vi "ReadSummaryResults.vi"(8 "error in (no error)":errorcluster, 11 "Path":path) -> (0 "error out":errorcluster, 3 "Results":dbl[][](array[numeric]))   [LabVIEW 2014]
uses:
  Excel(ActiveX)/enumOpenOrCreate.ctl
  Excel(ActiveX)/Excel(ActiveX).lvlib
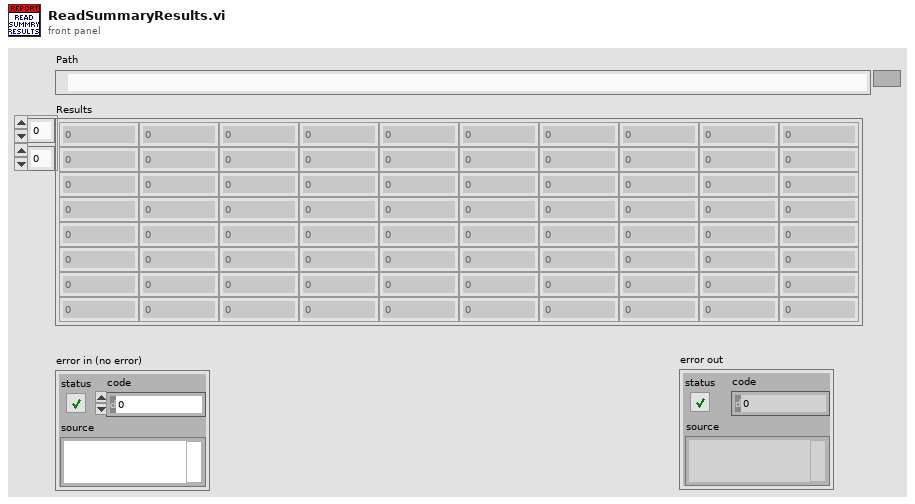
[diagram p1: front panel]
types:
  T1 = typedef "Excel(ActiveX).lvlib/enumOpenOrCreate.ctl" = enum16{"open", "open or create", "create from template"}
  T2 = typedef "Excel(ActiveX).lvlib/ExcelActiveX.ctl" = cluster{"Excel._Application":refnum<k7>, "Application open at start":bool, "Excel._Worksheet":refnum<k7>, "Workbook open at start":bool, "Excel._Workbook":refnum<k7>, "Workbook Path":path, "Worksheet Name":string, "Row":u32, "Col":u32, "Cell":string, "Workbook Name":string}
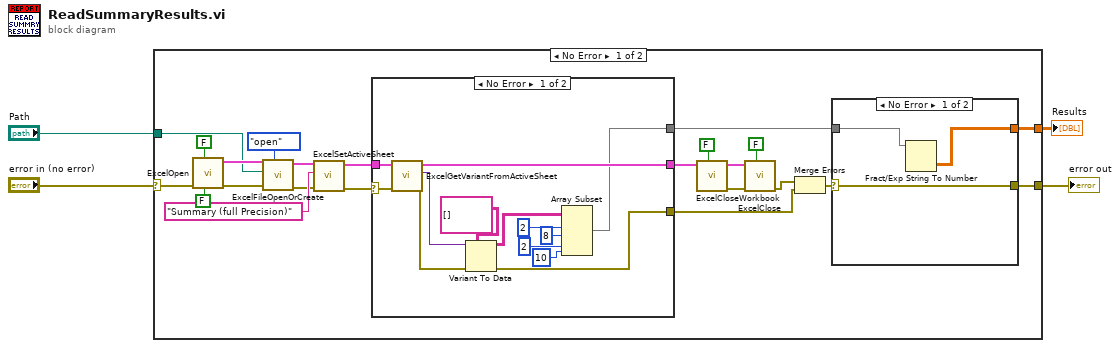
[diagram p0: block diagram]
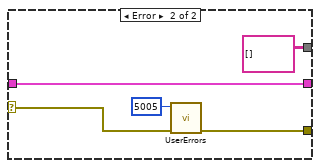
[diagram p2: hidden frame]
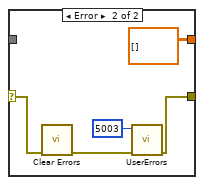
[diagram p3: hidden frame]
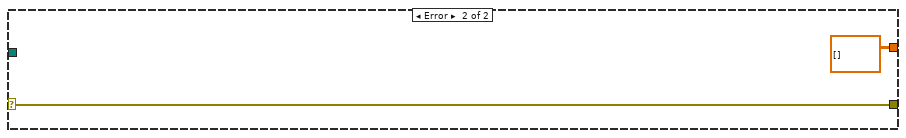
[diagram p4: hidden frame]
diagram:
  n1 = case shown="No Error" "error in (no error)" {
    selector: "error in (no error)" -> [w25 w55]
    tunnel: [w14 w55] -> w3
    tunnel: "Path" -> [w21 _]
    tunnel: [w9 dbl[][] []] -> w1
    frame No Error {
      n2 = call "ExcelOpen.vi"("Run Minimized (f)"=FALSE, "Excel visible? (t)"=FALSE, "error in (no error)"=w25) -> ("error out"=w23:errorcluster, "ExcelActiveX"=w22:T2)  [unwired: 7 in]
      n3 = call "ExcelFileOpenOrCreate.vi"("Open or Create"=enumOpenOrCreate."open", "error in (no error)"=w23, "Excel file name and path"=w21, "ExcelActiveX in"=w22) -> ("error out"=w19:errorcluster, "ExcelActiveX out"=w18:T2)  [unwired: 6 in]
      n4 = call "ExcelSetActiveSheet.vi"("error in (no error)"=w19, "Sheet Name"="Summary (full Precision)", "ExcelActiveX in"=w18) -> ("error out"=w11:errorcluster, "ExcelActiveX  out"=w13:T2)  [unwired: 7 in]
      n5 = case shown="No Error" w11 {
        selector: w11 -> [w38 w43]
        tunnel: w13 -> [w40 w45]
        tunnel: [w39 w45] -> w8
        tunnel: [w34 w42] -> w12
        tunnel: [w28 string[][] []] -> w10
        frame No Error {
          n6 = call "ExcelGetVariantFromActiveSheet.vi"("error in (no error)"=w38, "ExcelActiveX  in"=w40) -> ("error out"=w35:errorcluster, "VariantOut"=w37:variant, "ExcelActiveX  out"=w39:T2)  [unwired: 7 in]
          n7 = Variant To Data(error in=w35, type=string[][] [], Variant=w37) -> (data=w33:string[][], error out=w34:errorcluster)
          n8 = Array Subset(array=w33, index (row)=2 ("index"), length (row)=8 ("length"), index (col)=2 ("index"), length (col)=10 ("index")) -> (w28:string[][])
        }
        frame Error {
          n9 = call "UserErrors.vi"("error in (no error)"=w43, "[error code] (0)"=5005) -> ("error out"=w42:errorcluster)  [unwired: 9 in]
        }
      }
      n10 = call "ExcelCloseWorkbook.vi"("Save"=FALSE, "ExcelActiveX"=w8) -> ("error out"=w6:errorcluster, "ExcelActiveX"=w7:T2)  [unwired: 8 in]
      n11 = call "ExcelClose.vi"("Leave Open (f)"=FALSE, "error in (no error)"=w6, "ExcelActiveX in"=w7) -> ("error out"=w17:errorcluster)  [unwired: 7 in, 1 out]
      n12 = Merge Errors(w17, w12) -> (w15:errorcluster)
      n13 = case shown="No Error" w15 {
        selector: w15 -> [w48 w53]
        tunnel: [w48 w51] -> w14
        tunnel: w10 -> [w47 _]
        tunnel: [w46 dbl[][] []] -> w9
        frame No Error {
          n14 = Fract/Exp String To Number(string=w47) -> (number=w46:dbl[][])  [unwired: 3 in, 1 out]
        }
        frame Error {
          n15 = call <vilib>:"Clear Errors.vi"("error in (no error)"=w53) -> ("error out"=w52:errorcluster)  [unwired: 5 in, 1 out]
          n16 = call "UserErrors.vi"("error in (no error)"=w52, "[error code] (0)"=5003) -> ("error out"=w51:errorcluster)  [unwired: 9 in]
        }
      }
    }
    frame Error {
    }
  }
  "error out" <- w3
  "Results" <- w1
